vi "_Drivers Tree.vi"   [LabVIEW 2011]
uses:
  VNA/VNA Command.ctl
  PIM/PIM Command.ctl
  IMP/IMP Command.ctl
  SNA/SNA Command.ctl
panel:
  # "See Diagram"
types:
  T1 = typedef "SNA Command.ctl" = enum16{"LOAD", "INITIALIZE", "PRESET", "GET STIMULUS", "SET STIMULUS", "GET CALIBRATION", "CALIBRATE", "RESTORE", "MEASURE", "RELEASE", "UNLOAD", "CONFIRM", "SORT"}
  T2 = typedef "IMP Command.ctl" = enum16{"LOAD", "INITIALIZE", "IMPORT", "UNLOAD"}
  T3 = typedef "PIM Command.ctl" = enum16{"LOAD", "KEEP ALIVE", "VALIDATE", "INITIALIZE", "PRESET", "GET CALIBRATION", "SET STIMULUS", "TOGGLE TX POWER", "SET TX ON", "SET TX OFF", "MEASURE", "UNLOAD"}
  T4 = typedef "VNA Command.ctl" = enum16{"LOAD", "INITIALIZE", "PRESET", "GET STIMULUS", "SET STIMULUS", "GET CALIBRATION", "CALIBRATE", "RESTORE", "MEASURE", "RELEASE", "UNLOAD", "CONFIRM", "SORT"}
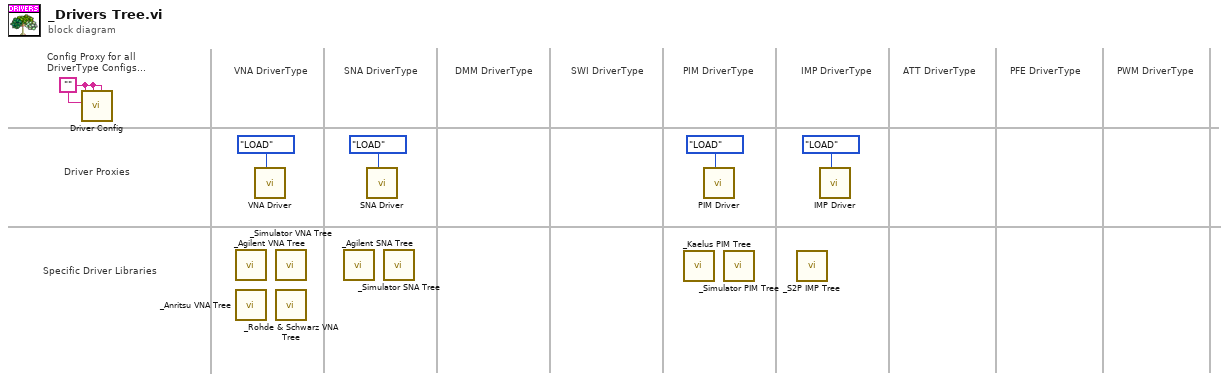
[diagram p0: block diagram]
diagram:
  w2 = ""
  # "PWM DriverType"
  # "PFE DriverType"
  # "ATT DriverType"
  # "SNA DriverType"
  # "IMP DriverType"
  # "PIM DriverType"
  # "SWI DriverType"
  # "DMM DriverType"
  # "Specific Driver Libraries"
  # "Driver Proxies"
  # "VNA DriverType"
  # "Config Proxy for all\nDriverType Configs..."
  n1 = call "Driver Config.vi"("DriverID (\"\")"=w2, "DriverType (\"\")"=w2, "Configuration In (Empty)"=w2, "TestStation Client (\"\")"=w2) -> ()  [unwired: 2 in, 6 out]
  n2 = call "_Agilent VNA Tree.vi"() -> ()  [unwired: 1 out]
  n3 = call "_Anritsu VNA Tree.vi"() -> ()  [unwired: 1 out]
  n4 = call "VNA Driver.vi"("VNA Command"=VNA_Command."LOAD") -> ()  [unwired: 6 in, 5 out]
  n5 = call "_Simulator VNA Tree.vi"() -> ()  [unwired: 1 out]
  n6 = call "_Rohde & Schwarz VNA Tree.vi"() -> ()  [unwired: 1 out]
  n7 = call "_Agilent SNA Tree.vi"() -> ()  [unwired: 1 out]
  n8 = call "SNA Driver.vi"("SNA Command"=SNA_Command."LOAD") -> ()  [unwired: 6 in, 5 out]
  n9 = call "_Simulator SNA Tree.vi"() -> ()  [unwired: 1 in]
  n10 = call "_Kaelus PIM Tree.vi"() -> ()  [unwired: 1 out]
  n11 = call "PIM Driver.vi"("PIM Command"=PIM_Command."LOAD") -> ()  [unwired: 4 in, 7 out]
  n12 = call "_Simulator PIM Tree.vi"() -> ()  [unwired: 1 in]
  n13 = call "_S2P IMP Tree.vi"() -> ()  [unwired: 1 out]
  n14 = call "IMP Driver.vi"("IMP Command"=IMP_Command."LOAD" ("VNA Command")) -> ()  [unwired: 4 in, 7 out]
